vi "Estimate total time.vi"(8 "error in (no error)":errorcluster, 11 "Tomo in":refnum<class "Tomo.lvclass">) -> (0 "error out":errorcluster, 2 "Total time":dbl[unit], 3 "Tomo out":refnum<class "Tomo.lvclass">)   [LabVIEW 2012, in "Tomo.lvclass"]
uses:
  Tomo.lvclass
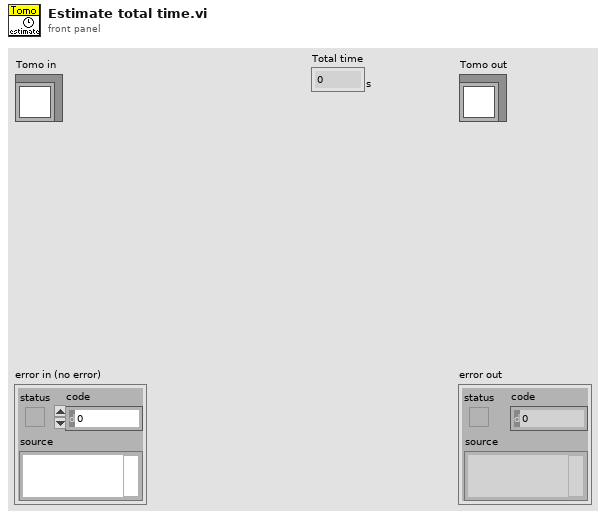
[diagram p1: front panel]
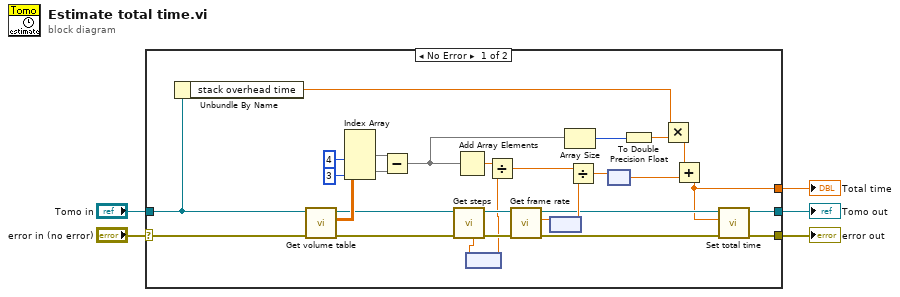
[diagram p0: block diagram]
diagram:
  n1 = case shown="No Error" "error in (no error)" {
    selector: "error in (no error)" -> [w34 w36]
    tunnel: [w17 w36] -> w4
    tunnel: [w15 w35] -> w2
    tunnel: "Tomo in" -> [w12 w35]
    tunnel: [w6 _] -> w1
    frame No Error {
      n2 = Unbundle By Name(w12) -> ("stack overhead time"=w11:dbl[unit])
      n3 = call-dynamic "Get volume table.vi"("error in (no error)"=w34, "Tomo in"=w12) -> ("error out"=w28:errorcluster, "Volume table out"=w33:dbl[][], "Tomo out"=w26:refnum<class "Tomo.lvclass">)  [unwired: 7 in]
      n4 = Index Array(array=w33, index (col) #1=4 ("disabled index (col)"), index (col) #2=3 ("index (col)")) -> (element #1=w30:dbl[], element #2=w29:dbl[])  [unwired: 2 in]
      n5 = Subtract(x=w30, y=w29) -> (x-y=w13:dbl[])
      n6 = call-dynamic "Get steps.vi"("error in (no error)"=w28, "Tomo in"=w26) -> ("error out"=w27:errorcluster, "Tomo out"=w25:refnum<class "Tomo.lvclass">, "Z step size"=w23:dbl[unit])  [unwired: 4 in, 3 out]
      n7 = Add Array Elements(numeric array=w13) -> (sum=w24:dbl)
      n8 = node(w23) -> (w20:dbl)
      n9 = Divide(x=w24, y=w20) -> (x/y=w21:dbl)
      n10 = call-dynamic "Get frame rate.vi"("error in (no error)"=w27, "Tomo in"=w25) -> ("error out"=w18:errorcluster, "Frame rate"=w22:dbl[unit], "Tomo out"=w16:refnum<class "Tomo.lvclass">)  [unwired: 7 in]
      n11 = node(w22) -> (w19:dbl)
      n12 = Array Size(array=w13) -> (size(s)=w10:i32)
      n13 = Divide(x=w21, y=w19) -> (x/y=w14:dbl)
      n14 = node(w14) -> (w7:dbl[unit])
      n15 = To Double Precision Float(number=w10) -> (double precision float=w9:dbl)
      n16 = Multiply(x=w11, y=w9) -> (x*y=w8:dbl[unit])
      n17 = Add(x=w8, y=w7) -> (x+y=w6:dbl[unit])
      n18 = call-dynamic "Set total time.vi"("error in (no error)"=w18, "Total time"=w6, "Tomo in"=w16) -> ("error out"=w17:errorcluster, "Tomo out"=w15:refnum<class "Tomo.lvclass">)  [unwired: 7 in]
    }
    frame Error {
    }
  }
  "error out" <- w4
  "Tomo out" <- w2
  "Total time" <- w1
